vi "Tree Config Data To Tree.vi"(6 "CFG Owning Path":path, 7 "Owning Tree":string, 8 "error in":errorcluster, 9 "Test Base Paths":T1[](array[typedef]), 10 "Test Config Data":T3[](array[typedef]) {"Test Ranking" items=["Low", "Normal", "High"]}, 11 "Tree Manager in":T2) -> (0 "error out":errorcluster, 3 "Tree Manager out":T2)   [LabVIEW 2020]
uses:
  <vilib>/addons/analyzer/_analyzerctrls.llb/VIAnCtl Test Config Data.ctl
  <vilib>/addons/analyzer/_analyzerctrls.llb/VIAnCtl TestRanking.ctl
  <vilib>/addons/analyzer/_analyzerctrls.llb/VIAnCtl Config Control Value.ctl
  <vilib>/addons/analyzer/VIAnCFGDataStructure/Tree Manager/Typedefs/Session Handle.ctl
  <vilib>/addons/analyzer/VIAnCFGDataStructure/Tree Manager/Tree.lvclass
  <vilib>/addons/analyzer/_vianuishared.llb/VIAnUI Test Base Path.ctl
  <vilib>/addons/analyzer/VIAnCFGDataStructure/Data Types/String/String.lvclass/String.ctl
  <vilib>/addons/analyzer/VIAnCFGDataStructure/Data Types/Int/Int.lvclass/Int.ctl
  <vilib>/addons/analyzer/VIAnCFGDataStructure/Data Types/Path/Path.lvclass/Path.ctl
  <vilib>/addons/analyzer/VIAnCFGDataStructure/Data Types/Bool/Bool.lvclass/Bool.ctl
  <vilib>/addons/analyzer/VIAnCFGDataStructure/Data Types/String Array/1D String.lvclass/1D String.ctl
  <vilib>/addons/analyzer/VIAnCFGDataStructure/Data Types/2D String/2D String.lvclass/2D String.ctl
  <vilib>/addons/analyzer/VIAnCFGDataStructure/Data Types/String/To String Tree Data.vi
  <vilib>/addons/analyzer/VIAnCFGDataStructure/Data Types/Bool/To Bool Tree Data.vi
  <vilib>/addons/analyzer/VIAnCFGDataStructure/Data Types/Path/To Path Tree Data.vi
  <vilib>/addons/analyzer/VIAnCFGDataStructure/Data Types/Int/To Integer Tree Data.vi
  <vilib>/addons/analyzer/VIAnCFGDataStructure/Data Types/String Array/To 1D String Tree Data.vi
  <vilib>/addons/analyzer/VIAnCFGDataStructure/Data Types/2D String/To 2D String Tree Data.vi
  <vilib>/addons/analyzer/VIAnCFGDataStructure/Data Types/String/String.lvclass
  e:/builds/penguin/labview/branches/2020/dev/dist/vi.lib/addons/analyzer/VIAnCFGDataStructure/Tree Data/Tree Data.lvclass
  <vilib>/addons/analyzer/VIAnCFGDataStructure/Data Types/Bool/Bool.lvclass
  <vilib>/addons/analyzer/VIAnCFGDataStructure/Data Types/Path/Path.lvclass
  <vilib>/addons/analyzer/VIAnCFGDataStructure/Data Types/Int/Int.lvclass
  <vilib>/addons/analyzer/VIAnCFGDataStructure/Data Types/String Array/1D String.lvclass
  <vilib>/addons/analyzer/VIAnCFGDataStructure/Data Types/2D String/2D String.lvclass
  <vilib>/addons/analyzer/VIAnCFGDataStructure/Data Types/Float/Flt.lvclass
  <vilib>/addons/analyzer/VIAnCFGDataStructure/Data Types/Int Array/1D Int.lvclass
  <vilib>/addons/analyzer/VIAnCFGDataStructure/Data Types/Flt Array/1D Flt.lvclass
  <vilib>/addons/analyzer/VIAnCFGDataStructure/Data Types/Bool Array/1D Bool.lvclass
  <vilib>/addons/analyzer/VIAnCFGDataStructure/Data Types/Path Array/1D Path.lvclass
  <vilib>/addons/analyzer/VIAnCFGDataStructure/Data Types/2D Int/2D Int.lvclass
  <vilib>/addons/analyzer/VIAnCFGDataStructure/Data Types/2D Flt/2D Flt.lvclass
  <vilib>/addons/analyzer/VIAnCFGDataStructure/Data Types/2D Bool/2D Bool.lvclass
  <vilib>/addons/analyzer/VIAnCFGDataStructure/Data Types/2D Path/2D Path.lvclass
  <vilib>/addons/analyzer/_vianuishared.llb/VIAnUI CFG File Info Global.vi
  <vilib>/addons/analyzer/VIAnCFGDataStructure/Tree Manager/API/Set Attribute Tree Data.vi
  <vilib>/Utility/error.llb/Error Cluster From Error Code.vi
  <vilib>/addons/analyzer/VIAnCFGDataStructure/Tree Data/Tree Data.lvclass
  e:/builds/penguin/labview/branches/2020/dev/dist/vi.lib/addons/analyzer/VIAnCFGDataStructure/Data Types/Int/Int.lvclass
  e:/builds/penguin/labview/branches/2020/dev/dist/vi.lib/addons/analyzer/VIAnCFGDataStructure/Data Types/String/String.lvclass
  <vilib>/Utility/Data Type/NI_Data Type.lvlib
  e:/builds/penguin/labview/branches/2020/dev/dist/vi.lib/addons/analyzer/VIAnCFGDataStructure/Data Types/Path/Path.lvclass
  e:/builds/penguin/labview/branches/2020/dev/dist/vi.lib/addons/analyzer/VIAnCFGDataStructure/Data Types/Bool/Bool.lvclass
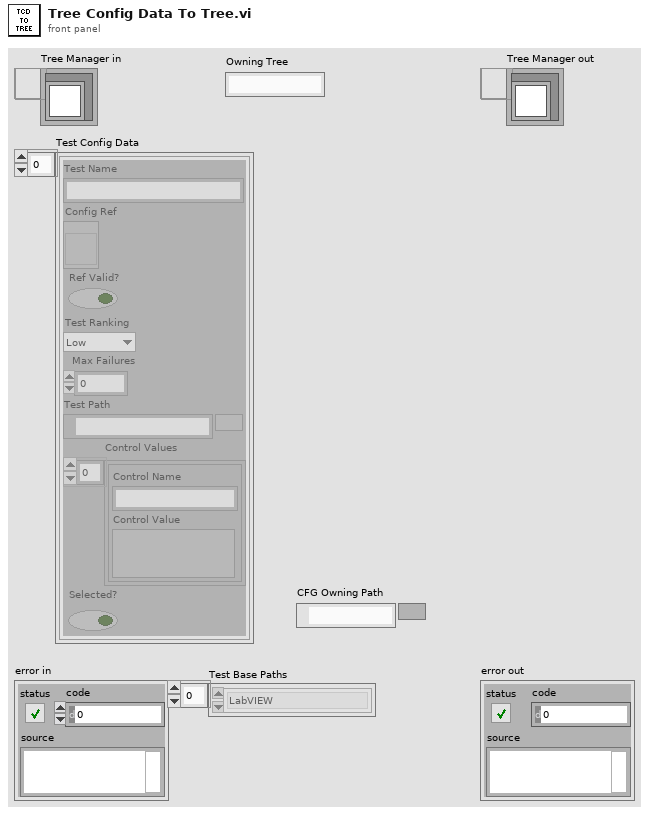
[diagram p1: front panel]
types:
  T1 = typedef "VIAnUI Test Base Path.ctl" = enum16{"LabVIEW", "LabVIEW Data"}
  T2 = typedef "NI_VIAnCFGDataStructure.lvlib/Tree.lvclass/Session Handle.ctl" = refnum<data-value>
  T3 = typedef "VIAnCtl Test Config Data.ctl" = cluster{"Test Name":string, "Config Ref":refnum<vi>, "Ref Valid?":bool, "Test Ranking":T4, "Max Failures":u32, "Test Path":path, "Control Values":T5[], "Selected?":bool}
  T4 = typedef "VIAnCtl TestRanking.ctl" = u16
  T5 = typedef "VIAnCtl Config Control Value.ctl" = cluster{"Control Name":string, "Control Value":variant}
  T6 = typedef "NI_Data Type.lvlib/Data Type.ctl" = enum8{"Invalid Type", "Void", "I8", "I16", "I32", "I64", "U8", "U16", "U32", "U64", "Single Float", "Double Float", "Extended Float", "Single Complex", "Double Complex", "Extended Complex", "Enum U8", "Enum U16", "Enum U32", "Enum U64", "Single Float With Unit", "Double Float With Unit", "Extended Float With Unit", "Single Complex with Unit", "Double Complex with Unit", "Extended Complex with Unit", "Boolean", "String", "Path", "Picture", "Tag", "Array", "Cluster", "Variant", "LV Variant", "Waveform", "Timestamp", "Digital Waveform", "Digital Data", "ExpressData", "Refnum", "External Data", "VI", "Poly VI", "LabVIEW Class Instance", "Fixed Point", "Set Collection", "Map Collection"}
  T7 = typedef "VIAnUI Path Type (viancfg).ctl" = enum16{"Relative", "RelativeToCFG", "RelativeToLabVIEW", "Network"}
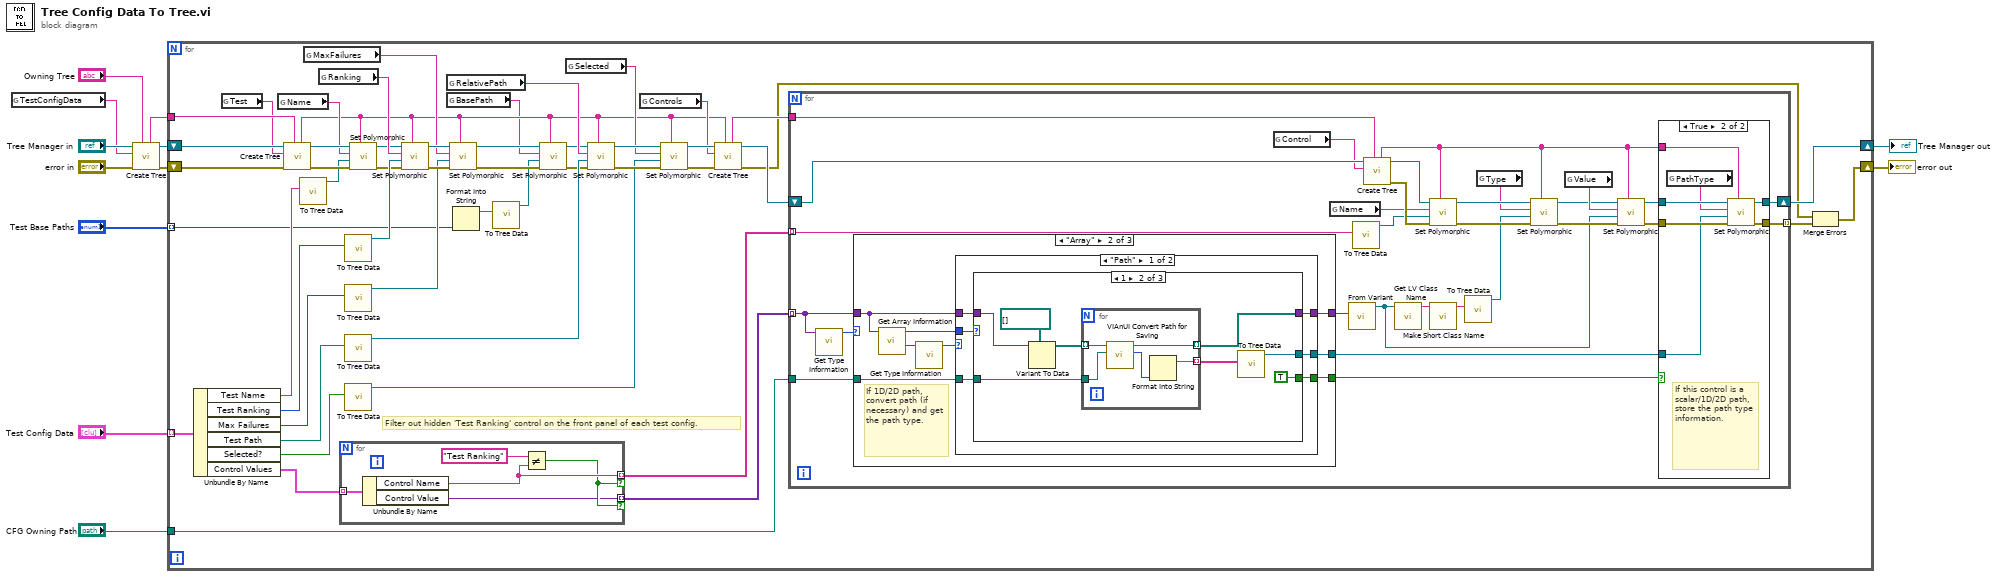
[diagram p0: block diagram]
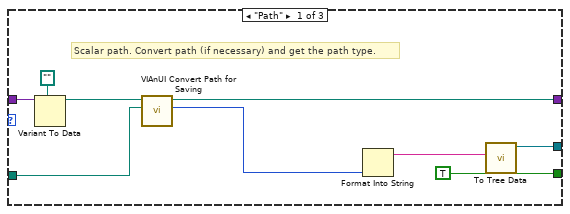
[diagram p2: hidden frame]
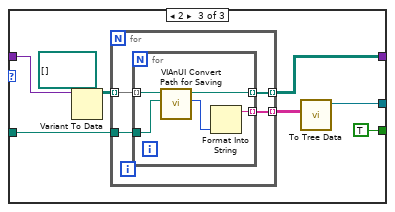
[diagram p4: hidden frame]
diagram:
  n1 = global read "VIAnUI CFG File Info Global.vi" "TestConfigData"() -> (w4:string)
  n2 = call <vilib>:"Create Tree.vi"("Parent ID (empty)"="Owning Tree", "Error In"="error in", "Name"=w4, "Tree Manager"="Tree Manager in") -> ("Error Out"=w8:errorcluster, "Tree Manager"=w9:T2, "Unique ID"=w7:string)  [unwired: 5 in]
  n3 = for {
    shift-right: [w57] -> w5
    shift-left: w9 -> [w60]
    shift-right: [w56] -> w11
    shift-left: w8 -> [w59]
    tunnel: "Test Config Data" -> [w62] mode=indexing
    tunnel: w7 -> [w61]
    tunnel: "Test Base Paths" -> [w17] mode=indexing
    tunnel: "CFG Owning Path" -> [w13]
    # "Filter out hidden 'Test Ranking' control on the front panel of each test config."
    n4 = Unbundle By Name(w62) -> ("Test Name"=w55:string, "Test Ranking"=w54:T4, "Max Failures"=w53:u32, "Test Path"=w52:path, "Selected?"=w51:bool, "Control Values"=w58:T5[])
    n5 = global read "VIAnUI CFG File Info Global.vi" "Test"() -> (w31:string)
    n6 = global read "VIAnUI CFG File Info Global.vi" "Name"() -> (w30:string)
    n7 = call <vilib>:"Create Tree.vi"("Parent ID (empty)"=w61, "Error In"=w59, "Name"=w31, "Tree Manager"=w60) -> ("Error Out"=w49:errorcluster, "Tree Manager"=w50:T2, "Unique ID"=w20:string)  [unwired: 5 in]
    n8 = call-poly <vilib>:"To Tree Data.vi"("String"=w55) -> ("String Tree Data"=w40:refnum<class "String.lvclass">)  [unwired: 10 in]
    n9 = global read "VIAnUI CFG File Info Global.vi" "MaxFailures"() -> (w28:string)
    n10 = global read "VIAnUI CFG File Info Global.vi" "Ranking"() -> (w29:string)
    n11 = for {
      tunnel: w58 -> [w67] mode=indexing
      tunnel: [w66] -> w35 mode=indexing if=w64
      tunnel: [w63] -> w34 mode=indexing if=w64
      n12 = Unbundle By Name(w67) -> ("Control Name"=w66:string, "Control Value"=w63:variant)
      n13 = Not Equal?(x="Test Ranking", y=w66) -> (x != y?=w64:bool)
    }
    n14 = call-poly <vilib>:"To Tree Data.vi"("Integer"=w54) -> ("Integer Tree Data"=w41:refnum<class "Int.lvclass">)  [unwired: 10 in]
    n15 = call-poly <vilib>:"To Tree Data.vi"("Integer"=w53) -> ("Integer Tree Data"=w42:refnum<class "Int.lvclass">)  [unwired: 10 in]
    n16 = call-poly <vilib>:"To Tree Data.vi"("Path"=w52) -> ("Path Tree Data"=w43:refnum<class "Path.lvclass">)  [unwired: 10 in]
    n17 = call-poly <vilib>:"To Tree Data.vi"("Boolean"=w51) -> ("Bool Tree Data"=w44:refnum<class "Bool.lvclass">)  [unwired: 10 in]
    n18 = call-poly <vilib>:"Set Polymorphic.vi"("Tree ID"=w20, "Error In"=w49, "Attribute Value"=w40, "Attribute Name"=w30, "Tree Manager"=w50) -> ("Error Out"=w23:errorcluster, "Tree Manager"=w24:T2)  [unwired: 4 in, 1 out]
    n19 = call-poly <vilib>:"Set Polymorphic.vi"("Tree ID"=w20, "Error In"=w23, "Attribute Value"=w41, "Attribute Name"=w29, "Tree Manager"=w24) -> ("Error Out"=w47:errorcluster, "Tree Manager"=w48:T2)  [unwired: 4 in, 1 out]
    n20 = global read "VIAnUI CFG File Info Global.vi" "RelativePath"() -> (w27:string)
    n21 = global read "VIAnUI CFG File Info Global.vi" "BasePath"() -> (w14:string)
    n22 = call-poly <vilib>:"Set Polymorphic.vi"("Tree ID"=w20, "Error In"=w47, "Attribute Value"=w42, "Attribute Name"=w28, "Tree Manager"=w48) -> ("Error Out"=w18:errorcluster, "Tree Manager"=w19:T2)  [unwired: 4 in, 1 out]
    n23 = Format Into String(w17) -> (resulting string=w16:string)  [unwired: 3 in, 1 out]
    n24 = call-poly <vilib>:"To Tree Data.vi"("String"=w16) -> ("String Tree Data"=w15:refnum<class "String.lvclass">)  [unwired: 10 in]
    n25 = call-poly <vilib>:"Set Polymorphic.vi"("Tree ID"=w20, "Error In"=w18, "Attribute Value"=w15, "Attribute Name"=w14, "Tree Manager"=w19) -> ("Error Out"=w21:errorcluster, "Tree Manager"=w22:T2)  [unwired: 4 in, 1 out]
    n26 = global read "VIAnUI CFG File Info Global.vi" "Selected"() -> (w26:string)
    n27 = call-poly <vilib>:"Set Polymorphic.vi"("Tree ID"=w20, "Error In"=w21, "Attribute Value"=w43, "Attribute Name"=w27, "Tree Manager"=w22) -> ("Error Out"=w45:errorcluster, "Tree Manager"=w46:T2)  [unwired: 4 in, 1 out]
    n28 = global read "VIAnUI CFG File Info Global.vi" "Controls"() -> (w25:string)
    n29 = call-poly <vilib>:"Set Polymorphic.vi"("Tree ID"=w20, "Error In"=w45, "Attribute Value"=w44, "Attribute Name"=w26, "Tree Manager"=w46) -> ("Error Out"=w38:errorcluster, "Tree Manager"=w39:T2)  [unwired: 4 in, 1 out]
    n30 = call <vilib>:"Create Tree.vi"("Parent ID (empty)"=w20, "Error In"=w38, "Name"=w25, "Tree Manager"=w39) -> ("Error Out"=w32:errorcluster, "Tree Manager"=w37:T2, "Unique ID"=w36:string)  [unwired: 5 in]
    n31 = for {
      shift-right: [w75] -> w57
      shift-left: w37 -> [w95]
      tunnel: w36 -> [w96]
      tunnel: w35 -> [w90] mode=indexing
      tunnel: w34 -> [w72] mode=indexing
      tunnel: [w76] -> w33 mode=indexing
      tunnel: w13 -> [w68]
      n32 = call <vilib>:"Get Type Information.vi"("variant"=w72) -> ("type"=w73:T6)  [unwired: 6 in, 4 out]
      n33 = case shown="\"Array\"" w73 {
        tunnel: w72 -> [w105 w111 w152]
        tunnel: [w102 w110 w152] -> w71
        tunnel: [w99 w106 _] -> w70
        tunnel: [TRUE w108 _] -> w69
        tunnel: w68 -> [w98 w107 _]
        frame "Path" {
          # "Scalar path. Convert path (if necessary) and get the path type."
          n34 = Variant To Data(type=path "", Variant=w105) -> (data=w103:path)  [unwired: 1 in, 1 out]
          n35 = call <vilib>:"VIAnUI Convert Path for Saving.vi"("CFG Path"=w98, "Path in"=w103) -> ("Path Type"=w101:T7, "Path out"=w102:path)  [unwired: 8 in]
          n36 = Format Into String(w101) -> (resulting string=w100:string)  [unwired: 3 in, 1 out]
          n37 = call-poly <vilib>:"To Tree Data.vi"("String"=w100) -> ("String Tree Data"=w99:refnum<class "String.lvclass">)  [unwired: 10 in]
        }
        frame "Array" {
          # "If 1D/2D path, convert path (if necessary) and get the path type."
          n38 = call <vilib>:"Get Array Information.vi"("variant"=w111) -> ("array element data type"=w113:variant, "number of dimensions"=w109:i32)  [unwired: 7 in, 2 out]
          n39 = call <vilib>:"Get Type Information.vi"("variant"=w113) -> ("type"=w112:T6)  [unwired: 6 in, 4 out]
          n40 = case shown="\"Path\"" w112 {
            tunnel: w111 -> [w118 w151]
            tunnel: [w117 w151] -> w110
            tunnel: w109 -> [w119 _]
            tunnel: [w116 _] -> w108
            tunnel: w107 -> [w115 _]
            tunnel: [w114 _] -> w106
            frame "Path" {
              n41 = case shown="1" w119 {
                tunnel: w118 -> [w120 w127 w140]
                tunnel: [w120 w123 w136] -> w117
                tunnel: [_ TRUE TRUE] -> w116
                tunnel: w115 -> [_ w124 w137]
                tunnel: [_ w121 w134] -> w114
                frame Default {
                  # "Unsupported number of dimensions"
                }
                frame 1 {
                  n42 = Variant To Data(type=path[] [], Variant=w127) -> (data=w125:path[])  [unwired: 1 in, 1 out]
                  n43 = for {
                    tunnel: w125 -> [w133] mode=indexing
                    tunnel: w124 -> [w132]
                    tunnel: [w130] -> w123 mode=indexing
                    tunnel: [w129] -> w122 mode=indexing
                    n44 = call <vilib>:"VIAnUI Convert Path for Saving.vi"("CFG Path"=w132, "Path in"=w133) -> ("Path Type"=w131:T7, "Path out"=w130:path)  [unwired: 8 in]
                    n45 = Format Into String(w131) -> (resulting string=w129:string)  [unwired: 3 in, 1 out]
                  }
                  n46 = call-poly <vilib>:"To Tree Data.vi"("1D String"=w122) -> ("1D String Tree Data"=w121:refnum<class "1D String.lvclass">)  [unwired: 10 in]
                }
                frame 2 {
                  n47 = Variant To Data(type=path[][] [], Variant=w140) -> (data=w138:path[][])  [unwired: 1 in, 1 out]
                  n48 = for {
                    tunnel: w138 -> [w145] mode=indexing
                    tunnel: w137 -> [w144]
                    tunnel: [w143] -> w136 mode=indexing
                    tunnel: [w142] -> w135 mode=indexing
                    n49 = for {
                      tunnel: w145 -> [w150] mode=indexing
                      tunnel: w144 -> [w149]
                      tunnel: [w147] -> w143 mode=indexing
                      tunnel: [w146] -> w142 mode=indexing
                      n50 = call <vilib>:"VIAnUI Convert Path for Saving.vi"("CFG Path"=w149, "Path in"=w150) -> ("Path Type"=w148:T7, "Path out"=w147:path)  [unwired: 8 in]
                      n51 = Format Into String(w148) -> (resulting string=w146:string)  [unwired: 3 in, 1 out]
                    }
                  }
                  n52 = call-poly <vilib>:"To Tree Data.vi"("2D String"=w135) -> ("2D String Tree Data"=w134:refnum<class "2D String.lvclass">)  [unwired: 10 in]
                }
              }
            }
            frame Default {
              # "Not an array of paths."
            }
          }
        }
        frame Default {
          # "Not a path or an array."
        }
      }
      n53 = global read "VIAnUI CFG File Info Global.vi" "Control"() -> (w94:string)
      n54 = global read "VIAnUI CFG File Info Global.vi" "Name"() -> (w91:string)
      n55 = call <vilib>:"From Variant.vi"("Variant"=w71) -> ("Tree Data Out"=w74:refnum<class "Tree Data.lvclass">)  [unwired: 9 in, 1 out]
      n56 = call-poly <vilib>:"To Tree Data.vi"("String"=w90) -> ("String Tree Data"=w89:refnum<class "String.lvclass">)  [unwired: 10 in]
      n57 = call <vilib>:"Create Tree.vi"("Parent ID (empty)"=w96, "Name"=w94, "Tree Manager"=w95) -> ("Error Out"=w93:errorcluster, "Tree Manager"=w92:T2, "Unique ID"=w77:string)  [unwired: 6 in]
      n58 = call <vilib>:"Get LV Class Name.vi"("object"=w74) -> ("class name"=w87:string)  [unwired: 9 in, 1 out]
      n59 = call-poly <vilib>:"Set Polymorphic.vi"("Tree ID"=w77, "Error In"=w93, "Attribute Value"=w89, "Attribute Name"=w91, "Tree Manager"=w92) -> ("Error Out"=w85:errorcluster, "Tree Manager"=w86:T2)  [unwired: 4 in, 1 out]
      n60 = call <vilib>:"Make Short Class Name.vi"("Class Name"=w87) -> ("Shortened Class Name"=w81:string)  [unwired: 10 in]
      n61 = call-poly <vilib>:"To Tree Data.vi"("String"=w81) -> ("String Tree Data"=w80:refnum<class "String.lvclass">)  [unwired: 10 in]
      n62 = global read "VIAnUI CFG File Info Global.vi" "Type"() -> (w82:string)
      n63 = call-poly <vilib>:"Set Polymorphic.vi"("Tree ID"=w77, "Error In"=w85, "Attribute Value"=w80, "Attribute Name"=w82, "Tree Manager"=w86) -> ("Error Out"=w84:errorcluster, "Tree Manager"=w83:T2)  [unwired: 4 in, 1 out]
      n64 = global read "VIAnUI CFG File Info Global.vi" "Value"() -> (w88:string)
      n65 = call-poly <vilib>:"Set Polymorphic.vi"("Tree ID"=w77, "Error In"=w84, "Attribute Value"=w74, "Attribute Name"=w88, "Tree Manager"=w83) -> ("Error Out"=w79:errorcluster, "Tree Manager"=w78:T2)  [unwired: 4 in, 1 out]
      n66 = case shown="True" w69 {
        tunnel: w79 -> [w154 w161]
        tunnel: w78 -> [w153 w160]
        tunnel: w77 -> [_ w159]
        tunnel: [w154 w158] -> w76
        tunnel: [w153 w157] -> w75
        tunnel: w70 -> [_ w155]
        frame False {
        }
        frame True {
          # "If this control is a scalar/1D/2D path, store the path type information."
          n67 = global read "VIAnUI CFG File Info Global.vi" "PathType"() -> (w156:string)
          n68 = call-poly <vilib>:"Set Polymorphic.vi"("Tree ID"=w159, "Error In"=w161, "Attribute Value"=w155, "Attribute Name"=w156, "Tree Manager"=w160) -> ("Error Out"=w158:errorcluster, "Tree Manager"=w157:T2)  [unwired: 4 in, 1 out]
        }
      }
    }
    n69 = Merge Errors(w32, w33) -> (w56:errorcluster)
  }
  "error out" <- w11
  "Tree Manager out" <- w5
